vi "delete Test.vi"(8 "error in (no error)":errorcluster caption="Fehler (Eingang, kein Fehler)", 10 "id":i32, 11 "Test Eingang":refnum<class "Norm.lvclass"> caption="DNL_LabVIEW Object in") -> (0 "error out":errorcluster caption="Fehler (Ausgang)", 3 "Test Ausgang":refnum<class "Norm.lvclass"> caption="DNL_LabVIEW Object out")   [LabVIEW 2013, in "DatenKlassen.lvlib" / "Norm.lvclass"]
uses:
  Norm.lvclass
  Norm.lvclass/Norm.ctl
  Test/Test.lvclass
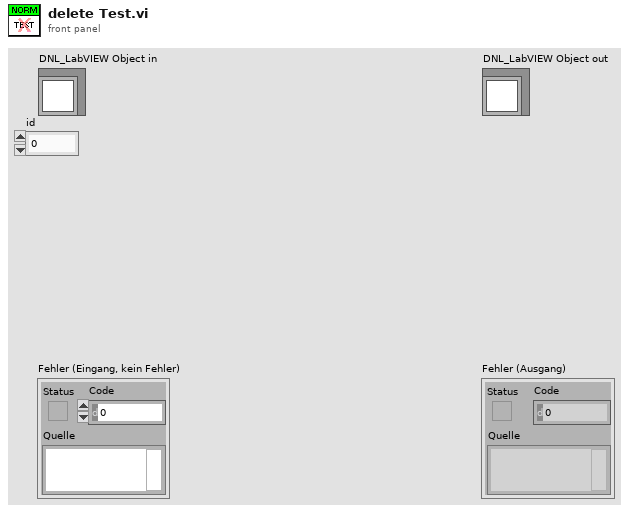
[diagram p1: front panel]
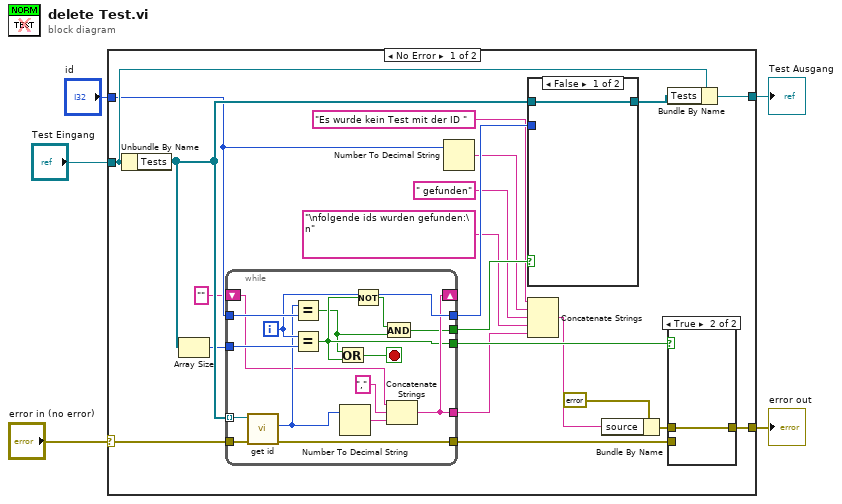
[diagram p0: block diagram]
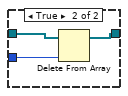
[diagram p2: hidden frame]
diagram:
  n1 = case shown="No Error" "error in (no error)" {
    selector: "error in (no error)" -> [w12 w50]
    tunnel: [w10 w50] -> w4
    tunnel: [w9 w49] -> w2
    tunnel: "Test Eingang" -> [w13 w49]
    tunnel: "id" -> [w11 _]
    frame No Error {
      n2 = Unbundle By Name(w13) -> ("Tests"=w24:refnum<class "Test.lvclass">[])
      n3 = Array Size(array=w24) -> (size(s)=w14:i32)
      n4 = while {
        tunnel: w24 -> [w44] mode=indexing
        tunnel: w11 -> [w48]
        tunnel: w14 -> [w47]
        tunnel: [w36] -> w20
        tunnel: [w33] -> w22
        tunnel: [w42] -> w23
        tunnel: w12 -> [w45]
        tunnel: [w43] -> w26
        shift-right: [w37] -> _
        shift-left: "" -> [w38]
        tunnel: [w37] -> w7
        i -> [w42]
        stop <- w46 stop-if-true
        n5 = call-dynamic "get id.vi"("error in (no error)"=w45, "Test in"=w44) -> ("error out"=w43:errorcluster, "id"=w41:u32)  [unwired: 7 in, 1 out]
        n6 = Equal?(x=w41, y=w48) -> (x = y?=w34:bool)
        n7 = Equal?(x=w42, y=w47) -> (x = y?=w36:bool)
        n8 = Or(x=w34, y=w36) -> (x .or. y?=w46:bool)
        n9 = Number To Decimal String(number=w41) -> (decimal integer string=w39:string)  [unwired: 1 in]
        n10 = Not(x=w36) -> (.not. x?=w35:bool)
        n11 = And(x=w35, y=w34) -> (x .and. y?=w33:bool)
        n12 = Concatenate Strings(w38, "," ("string"), w39) -> (w37:string)
      }
      n13 = Number To Decimal String(number=w11) -> (decimal integer string=w16:string)  [unwired: 1 in]
      n14 = case shown="False" w22 {
        tunnel: w23 -> [_ w29]
        tunnel: w24 -> [w27 w30]
        tunnel: [w27 w28] -> w25
        frame False {
        }
        frame True {
          n15 = Delete From Array(array=w30, index=w29) -> (array with subset deleted=w28:refnum<class "Test.lvclass">[])  [unwired: 1 in, 1 out]
        }
      }
      n16 = Concatenate Strings("Es wurde kein Test mit der ID " ("source"), w16, " gefunden" ("string"), "\nfolgende ids wurden gefunden:\n" ("string"), w7) -> (w19:string)
      n17 = Bundle By Name(cluster=errorcluster {"status"=TRUE, "code"=99999, "source"="Es wurde keine Norm mit der ID "} ("error constant"), "source"=w19) -> (w21:errorcluster)
      n18 = Bundle By Name(cluster=w13, "Tests"=w25) -> (w9:refnum<class "Norm.lvclass">)
      n19 = case shown="True" w20 {
        tunnel: [w31 w32] -> w10
        tunnel: w21 -> [_ w32]
        tunnel: w26 -> [w31 _]
        frame False {
        }
        frame True {
        }
      }
    }
    frame Error {
    }
  }
  "error out" <- w4
  "Test Ausgang" <- w2
